vi "Read Encryption.vi"(11 "ConfigManager in":refnum<class "ConfigManager.lvclass">) -> (2 "Encryption":refnum<class "Encryption.lvclass">, 3 "ConfigManager out":refnum<class "ConfigManager.lvclass">)   [LabVIEW 2013, in "CfgManager.lvlib" / "ConfigManager.lvclass"]
uses:
  ConfigManager.lvclass
  Encryption/Encryption.lvclass
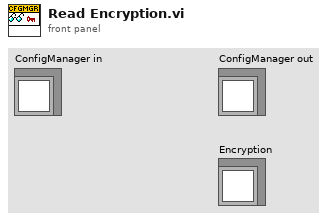
[diagram p1: front panel]
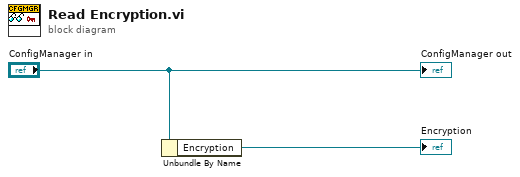
[diagram p0: block diagram]
diagram:
  n1 = Unbundle By Name("ConfigManager in") -> ("Encryption"=→"Encryption":refnum<class "Encryption.lvclass">)
  "ConfigManager out" <- "ConfigManager in"
